vi "CRYReport Unflatten.vi"(11 "Flatten Report":string) -> (0 "Error?":bool=TRUE, 2 "Checked Flatten Report":string, 3 "Header info":T1={"Data type"="Data            ", "Version"=1, "Dimensions"=0})   [LabVIEW 2013]
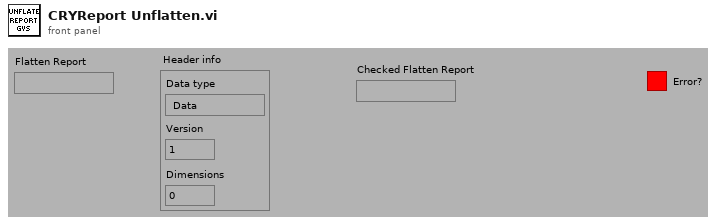
[diagram p1: front panel]
types:
  T1 = cluster{"Data type":string, "Version":u16, "Dimensions":u8}
  T2 = cluster{"cPages":cluster{"nPage":i32, "sTitle":string, "sIcon":string, "pVI":refnum<vi>, "nID":i32}[], "pTab":refnum<vi>, "nIDPages":i32[], "nStatID":i32}[]
  T3 = cluster{"unsigned byte array[0]":u8, "unsigned byte array[1]":u8, "unsigned byte array[2]":u8}
  T4 = cluster{"substring":string, u16, "unsigned byte array[2]":u8}
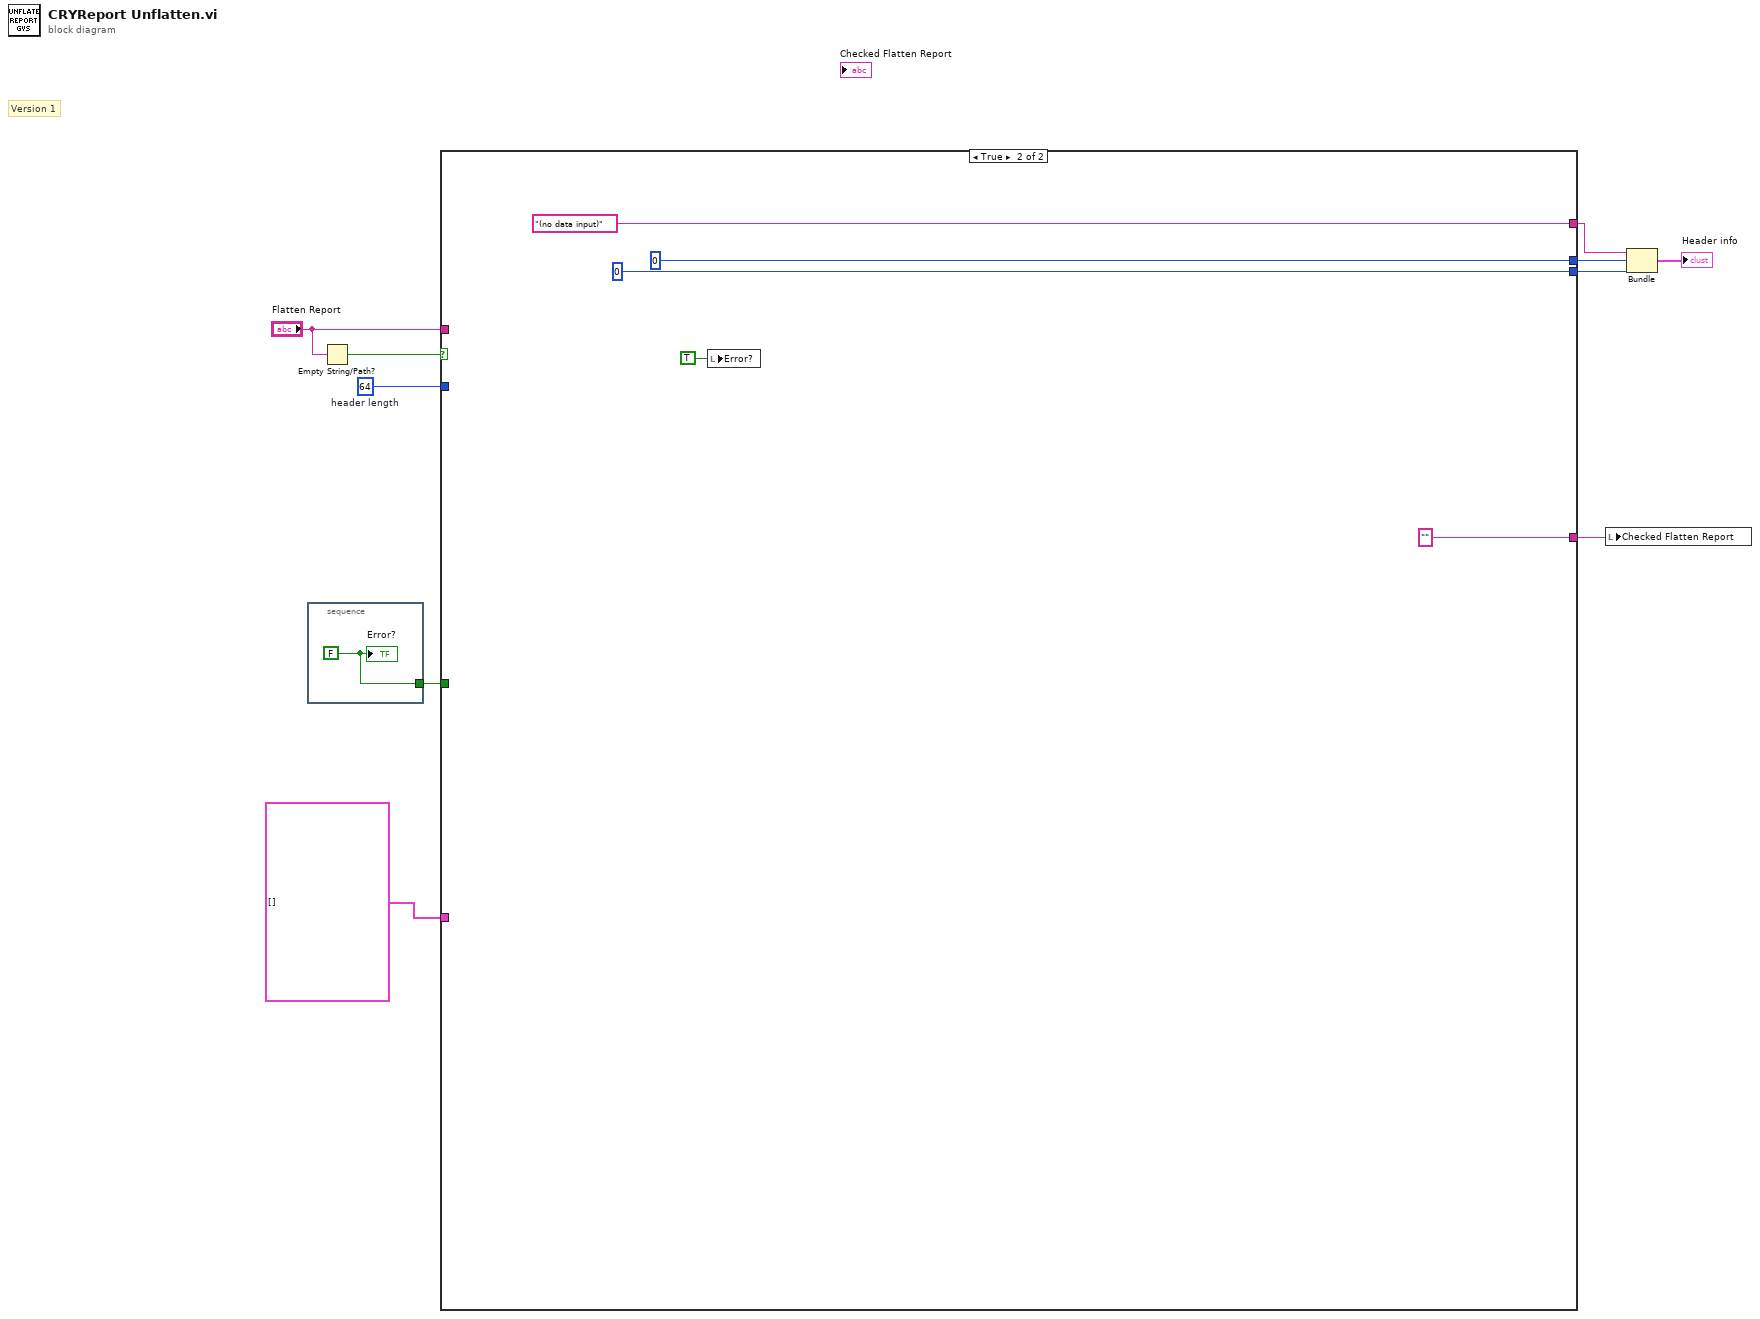
[diagram p0: block diagram]
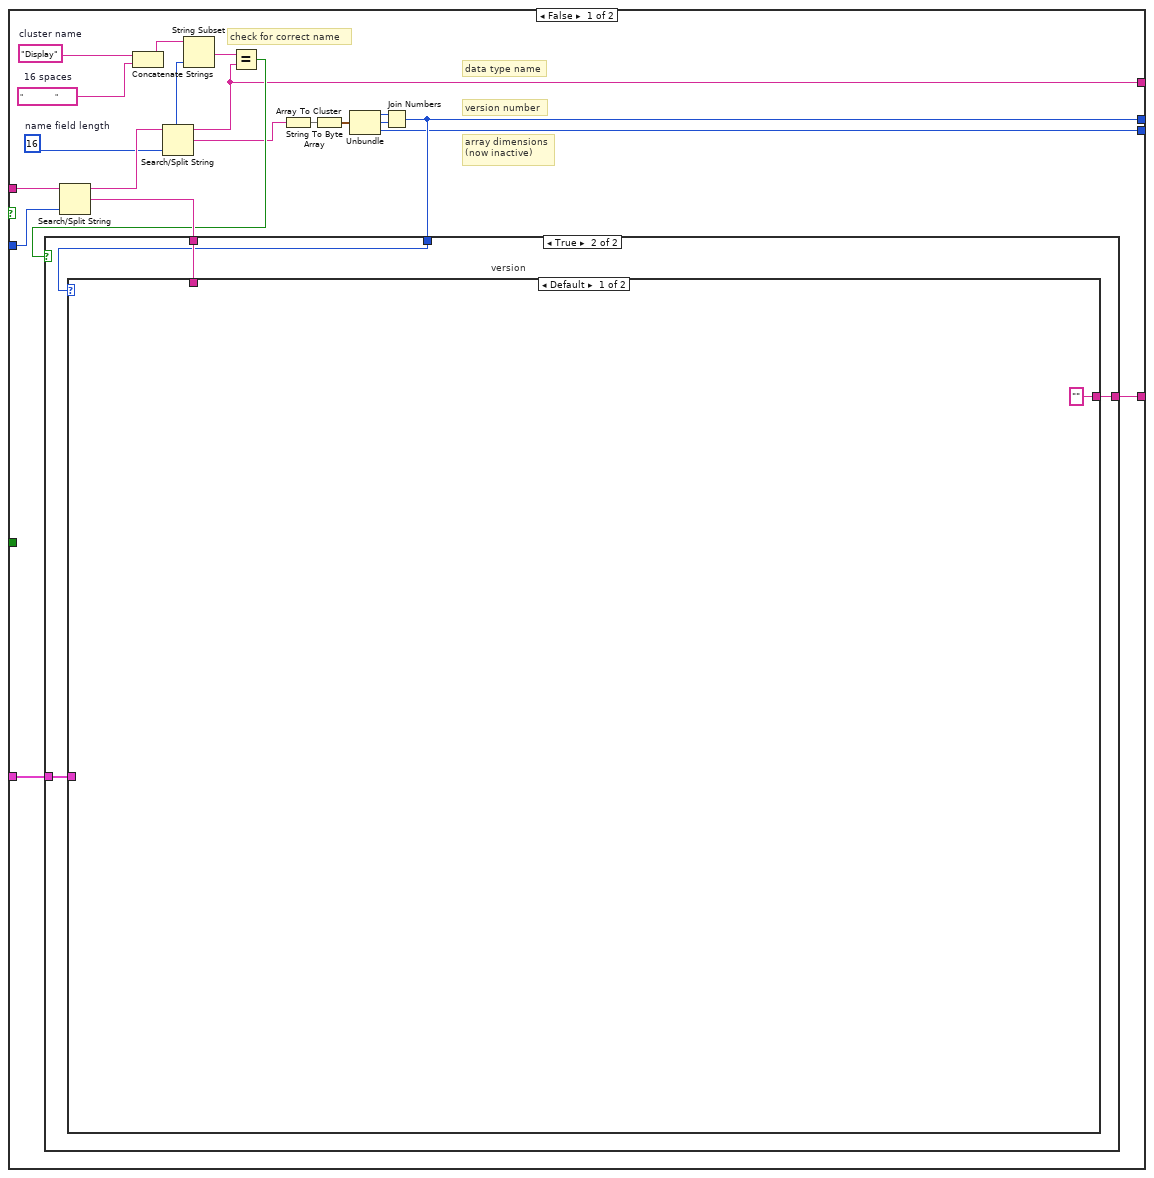
[diagram p2: hidden frame]
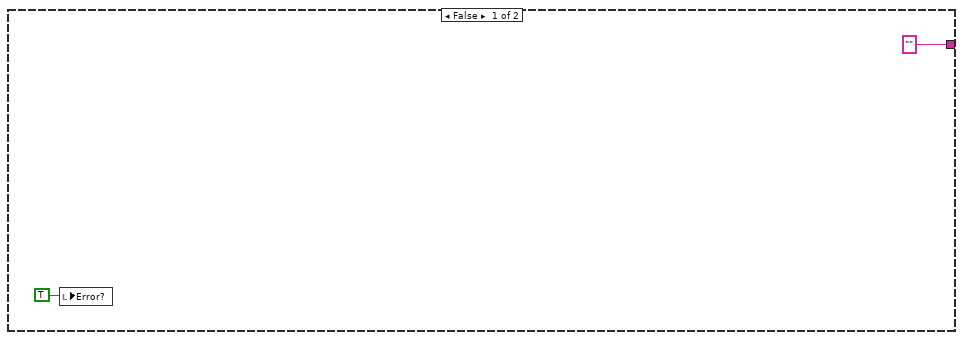
[diagram p3: hidden frame]
diagram:
  w9 = 64  # header length
  # "Version 1"
  n1 = stacked-sequence {
    tunnel: [w11] -> w4
    frame #0 {
      w11 = FALSE
      "Error?" <- w11
    }
  }
  n2 = Empty String/Path?(string/path="Flatten Report") -> (empty?=w10:bool)
  n3 = case shown="True" w10 {
    tunnel: "Flatten Report" -> [w31 _]
    tunnel: w9 -> [w25 _]
    tunnel: [w22 u16 0] -> w7
    tunnel: [w14 u8 0] -> w8
    tunnel: [w15 "(no data input)" ("substring")] -> w6
    tunnel: w4 -> [_ _]
    tunnel: T2 [] ("TabArray") -> [w13 _]
    tunnel: [w12 "" ("Flatten Report")] -> w1
    frame False {
      w19 = "                "  # 16 spaces
      w20 = "Display"  # cluster name
      w17 = 16  # name field length
      # "check for correct name"
      # "array dimensions\n(now inactive)"
      # "version number"
      # "data type name"
      n4 = Search/Split String(string=w31, offset (0)=w25) -> (substring before match=w24:string, match + rest of string=w26:string)  [unwired: 2 out]
      n5 = Concatenate Strings(w20, w19) -> (w18:string)
      n6 = Search/Split String(string=w24, offset (0)=w17) -> (substring before match=w15:string, match + rest of string=w21:string)  [unwired: 2 out]
      n7 = String Subset(string=w18, length (rest)=w17) -> (substring=w16:string)  [unwired: 1 out]
      n8 = Equal?(x=w16, y=w15) -> (x = y?=w23:bool)
      n9 = String To Byte Array(string=w21) -> (unsigned byte array=w30:u8[])
      n10 = Array To Cluster(array=w30) -> (cluster=w29:T3)
      n11 = Unbundle(w29) -> ("unsigned byte array[0]"=w28:u8, "unsigned byte array[1]"=w27:u8, "unsigned byte array[2]"=w14:u8)
      n12 = Join Numbers(hi=w28, lo=w27) -> ((hi.lo)=w22:u16)
      n13 = case shown="True" w23 {
        tunnel: w26 -> [_ w37]
        tunnel: w22 -> [_ w36]
        tunnel: w13 -> [_ w35]
        tunnel: ["" w34] -> w12
        frame False {
          n14 = local write "Error?"(TRUE) -> ()
        }
        frame True {
          n15 = case "version" shown="Default" w36 {
            tunnel: w37 -> [_ w39]
            tunnel: w35 -> [_ _]
            tunnel: ["" ("Flatten Report") w39] -> w34
            frame Default {
            }
            frame 1 {
            }
          }
        }
      }
    }
    frame True {
      n16 = local write "Error?"(TRUE ("Error?")) -> ()
    }
  }
  n17 = local write "Checked Flatten Report"(w1) -> ()
  n18 = Bundle("substring"=w6, w7, "unsigned byte array[2]"=w8) -> (→"Header info":T4)  [unwired: 1 out]
